vi "Get HPS Fault Code Info.vi"(11 "fault code":u64=3892314123 format="%08x") -> (1 "CLIP error bits":i32[](array[numeric]), 2 "fault enums":T1[](array[typedef]) items=["ERROR_GLOB_EMO_GLOBAL"=0, "ERROR_GLOB_EMO_BUTTON_PRESSED"=1, "ERROR_GLOB_USER"=2, "ERROR_GLOB_PM"=3, "ERROR_GLOB_GRID"=4, "ERROR_GLOB_VOLTAGE_DCBUS_OUT_OF_BOUNDS"=6, "ERROR_GLOB_VOLTAGE_OUTPUT_HIGH"=7, "ERROR_GLOB_VOLTAGE_OUTPUT_LOW"=8, "ERROR_GLOB_VOLTAGE_OUTPUT_UNBALANCE"=9, "ERROR_GLOB_CURRENT_OUTPUT_HIGH"=10, "ERROR_GLOB_SYS_OVERTEMPERATURE"=13, "ERROR_GLOB_SYS_HW"=14, "ERROR_GLOB_SYS_COMM"=15, "ERROR_GLOB_SYNC_AND_CONNECT"=16, "ERROR_GLOB_SP"=20, "ERROR_GLOB_SP_TRACKING"=21, "ERROR_GLOB_CONFIG"=23, "ERROR_GLOB_REG_SYS"=27, "ERROR_GLOB_REG_GRID"=28, "ERROR_GLOB_REG_AFE1"=29, "ERROR_GLOB_REG_AFE2"=30, "ERROR_GLOB_REG_DC"=31], 3 "is fault?":bool)   [LabVIEW 2023, in "HPS-17000-PowerModule.lvlib" / "HPS-17000-PowerModule.lvclass"]
uses:
  HPS-17000-PowerModule.lvclass
  ERROR_GLOBAL.ctl
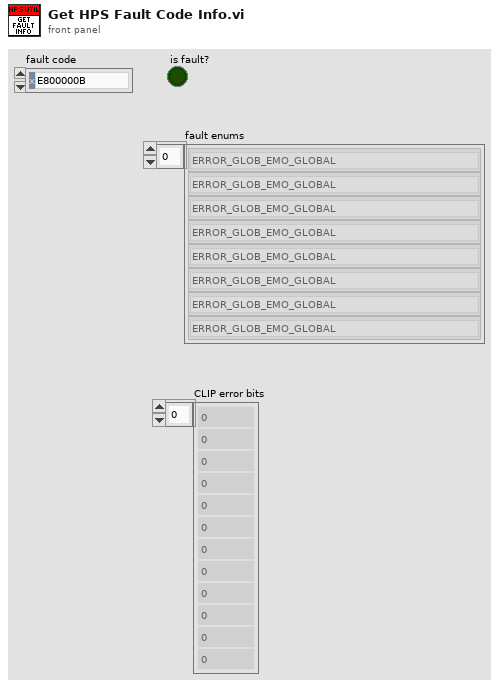
[diagram p1: front panel]
types:
  T1 = typedef "HPS-17000-PowerModule.lvlib/HPS-17000-PowerModule.lvclass/ERROR_GLOBAL.ctl" = u32
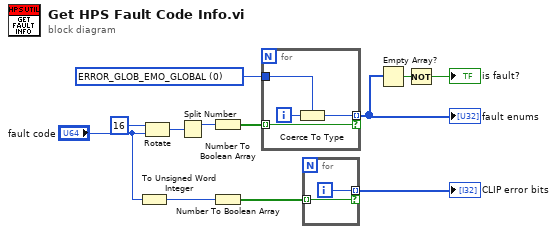
[diagram p0: block diagram]
diagram:
  w12 = T1 0 items=["ERROR_GLOB_EMO_GLOBAL"=0, "ERROR_GLOB_EMO_BUTTON_PRESSED"=1, "ERROR_GLOB_USER"=2, "ERROR_GLOB_PM"=3, "ERROR_GLOB_GRID"=4, "ERROR_GLOB_VOLTAGE_DCBUS_OUT_OF_BOUNDS"=6, "ERROR_GLOB_VOLTAGE_OUTPUT_HIGH"=7, "ERROR_GLOB_VOLTAGE_OUTPUT_LOW"=8, "ERROR_GLOB_VOLTAGE_OUTPUT_UNBALANCE"=9, "ERROR_GLOB_CURRENT_OUTPUT_HIGH"=10, "ERROR_GLOB_SYS_OVERTEMPERATURE"=13, "ERROR_GLOB_SYS_HW"=14, "ERROR_GLOB_SYS_COMM"=15, "ERROR_GLOB_SYNC_AND_CONNECT"=16, "ERROR_GLOB_SP"=20, "ERROR_GLOB_SP_TRACKING"=21, "ERROR_GLOB_CONFIG"=23, "ERROR_GLOB_REG_SYS"=27, "ERROR_GLOB_REG_GRID"=28, "ERROR_GLOB_REG_AFE1"=29, "ERROR_GLOB_REG_AFE2"=30, "ERROR_GLOB_REG_DC"=31] ("ERROR_GLOBAL")
  n1 = To Unsigned Word Integer(number="fault code") -> (unsigned 16bit integer=w2:u16)
  n2 = Rotate(1:"fault code", 2:i16 16 ("y")) -> (0:w6:u64)
  n3 = Split Number(x=w6) -> (hi(x)=w4:u32)  [unwired: 1 out]
  n4 = Number To Boolean Array(number=w4) -> (Boolean array=w3:bool[])
  n5 = Number To Boolean Array(number=w2) -> (Boolean array=w1:bool[])
  n6 = for {
    tunnel: w3 -> [w13] mode=indexing
    tunnel: w12 -> [w15]
    tunnel: [w14] -> w9 mode=indexing if=w13
    i -> [w16]
    n7 = Coerce To Type(0:w16, 1:w15) -> (2:w14:T1)
  }
  "fault enums" <- w9
  n8 = for {
    tunnel: w1 -> [w18] mode=indexing
    tunnel: [w17] -> w8 mode=indexing if=w18
    i -> [w17]
  }
  "CLIP error bits" <- w8
  n9 = Empty Array?(array=w9) -> (empty?=w11:bool)
  n10 = Not(x=w11) -> (.not. x?=→"is fault?":bool)
